vi "DetectCollision.vi"(9 "enemy_robots":T1[](array[typedef]), 10 "Point":dbl[](array[numeric])) -> (2 "Collision":bool)   [LabVIEW 2017]
uses:
  Core/AI Robot.ctl
  Intel/Functions Enum.ctl
  Intel/AttackerStates.ctl
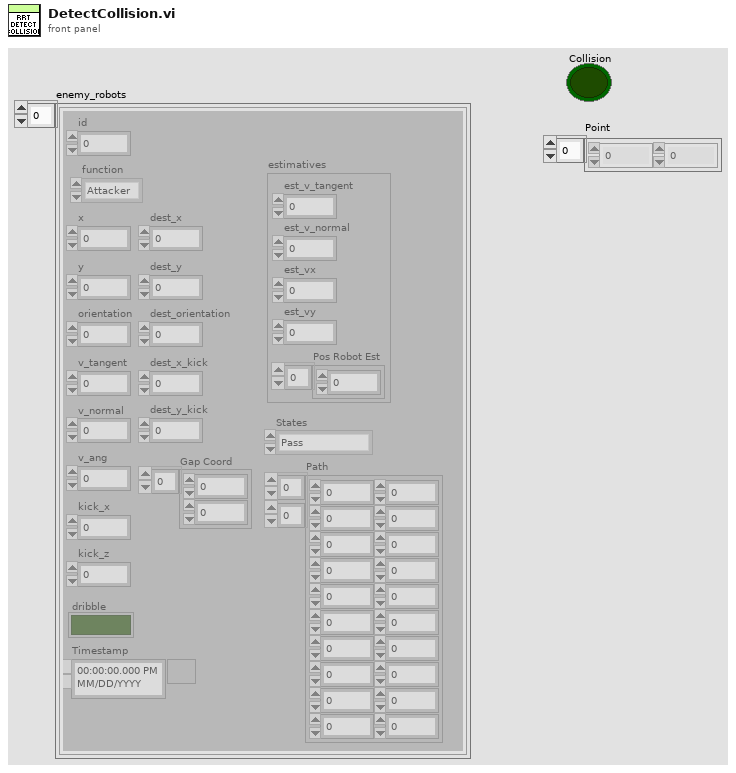
[diagram p1: front panel]
types:
  T1 = typedef "AI Robot.ctl" = cluster{"id":u32, "function":T2, "x":dbl, "y":dbl, "orientation":dbl, "v_tangent":dbl, "v_normal":dbl, "v_ang":dbl, "kick_x":dbl, "kick_z":dbl, "dribble":bool, "Timestamp":timestamp, "dest_x":dbl, "dest_y":dbl, "dest_orientation":dbl, "estimatives":cluster{"est_v_tangent":dbl, "est_v_normal":dbl, "est_vx":dbl, "est_vy":dbl, "Pos Robot Est":dbl[]}, "dest_x_kick":dbl, "dest_y_kick":dbl, "Gap Coord":dbl[], "States":T3, "Path ":dbl[][]}
  T2 = typedef "Functions Enum.ctl" = enum16{"Attacker", "Goalie", "Defender", "Striker", "Goto 0", "Dummy", "Kicker", "ZigZag"}
  T3 = typedef "AttackerStates.ctl" = enum16{"Pass", "GoToTangent", "BallGetting", "GoToKick", ""}
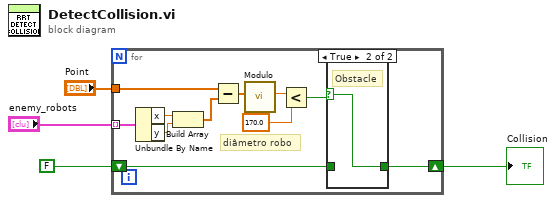
[diagram p0: block diagram]
diagram:
  n1 = for {
    tunnel: "enemy_robots" -> [w15] mode=indexing
    tunnel: "Point" -> [w11]
    shift-right: [w5] -> w1
    shift-left: FALSE -> [w6]
    # "diâmetro robo"
    n2 = Unbundle By Name(w15) -> ("x"=w14:dbl, "y"=w13:dbl)
    n3 = Build Array(w14, w13) -> (w12:dbl[])
    n4 = Subtract(x=w11, y=w12) -> (x-y=w10:dbl[])
    n5 = call "Modulo.vi"("2D vector"=w10) -> ("Modulo"=w9:dbl)  [unwired: 10 in]
    n6 = Less?(x=w9, y=170.0) -> (x < y?=w7:bool)
    n7 = case shown="True" w7 {
      selector: w7 -> [_ w17]
      tunnel: w6 -> [w16 _]
      tunnel: [w16 w17] -> w5
      frame False {
      }
      frame True {
        # "Obstacle"
      }
    }
  }
  "Collision" <- w1
